vi "Get_JSON_data.vi"(13 "detection":T1(array[cluster]), 14 "index\n detections":i32) -> (2 "element":T2, 4 "Coordonnées\n Rectangles":dbl[](array[numeric]), 6 "crop_path":string, 8 "confidence":i32, 10 "detection_type":string, 15 "label":string)   [LabVIEW 2024]
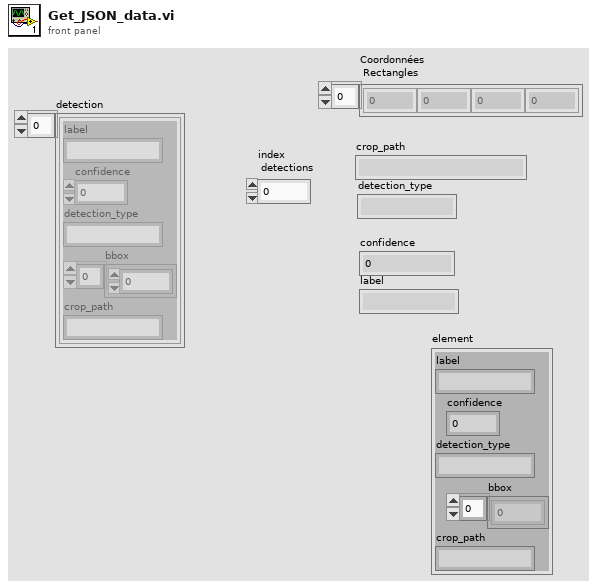
[diagram p1: front panel]
types:
  T1 = cluster{"label":string, "confidence":i32, "detection_type":string, "bbox":dbl[], "crop_path":string}[]
  T2 = cluster{"label":string, "confidence":i32, "detection_type":string, "bbox":dbl[], "crop_path":string}
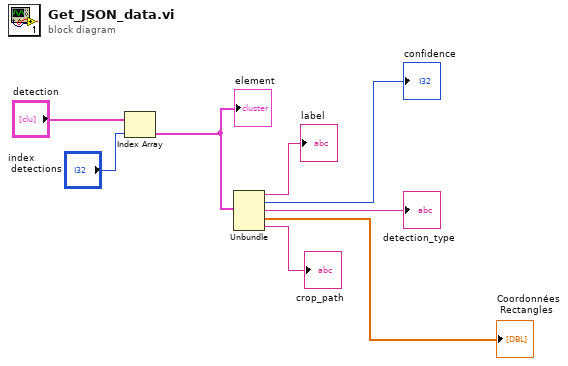
[diagram p0: block diagram]
diagram:
  n1 = Index Array(array="detection", index="index\n detections") -> (element=w7:T2)
  "element" <- w7
  n2 = Unbundle(w7) -> ("label"=→"label":string, "confidence"=→"confidence":i32, "detection_type"=→"detection_type":string, "bbox"=→"Coordonnées\n Rectangles":dbl[], "crop_path"=→"crop_path":string)
